vi "test error.vi"(8 "error in (no error)":errorcluster, 11 "VI Tester Test in":refnum<class "VI Tester Test 11.lvclass">=refnum) -> (0 "error out":errorcluster, 3 "VI Tester Test out":refnum<class "VI Tester Test 11.lvclass">)   [LabVIEW 2020, in "VI Tester Test 11.lvclass"]
uses:
  VI Tester Test 11.lvclass
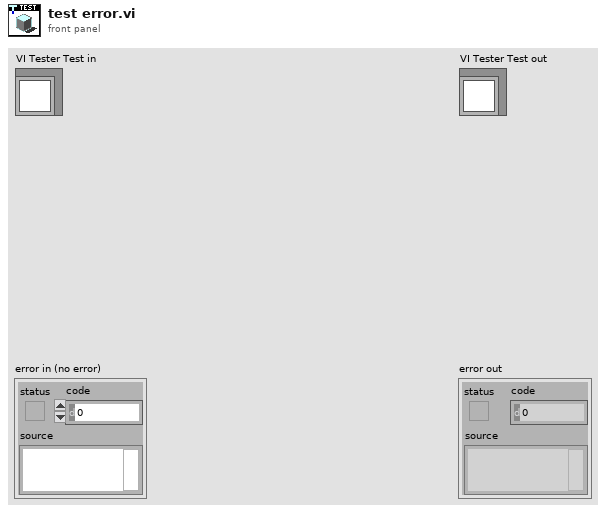
[diagram p1: front panel]
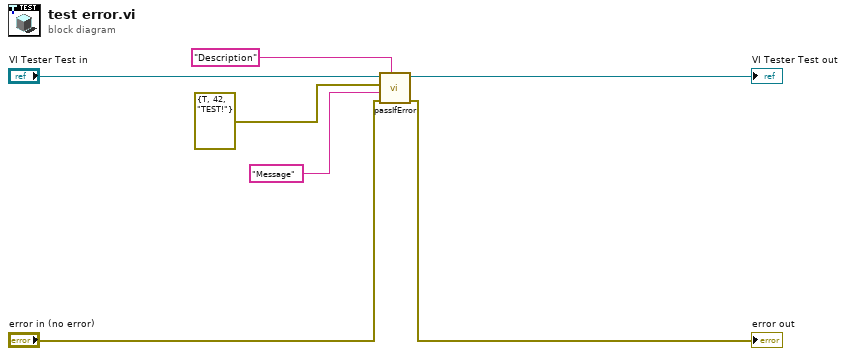
[diagram p0: block diagram]
diagram:
  n1 = call-dynamic "passIfError.vi"("custom report message (\"\")"="Description" ("Description"), "error in (no error)"="error in (no error)", "task (\"\")"="Message" ("task (\"\")"), "error"=errorcluster {"status"=TRUE, "code"=42, "source"="TEST!"} ("error in (no error)"), "TestCase in"="VI Tester Test in") -> ("error out"=→"error out":errorcluster, "TestCase out"=→"VI Tester Test out":refnum<class "VI Tester Test 11.lvclass">)  [unwired: 5 in]
